vi "Smite.vi"(4 "Hook Search Path":path[](array[path]), 6 "Execute Hooks?":cluster{"Pre":bool, "Post":bool}={"Pre"=TRUE, "Post"=TRUE}, 8 "Error In":errorcluster, 10 "Graves":refnum<vi>[](array[refnum]), 11 "VI In":refnum<vi>) -> (0 "Error Out":errorcluster, 2 "Change Made?":bool, 3 "VI Out":refnum<vi>)   [LabVIEW 2018, in "Toolkit.lvlib"]
doc: "Changes zombies back into corpses at each grave. Disables the Corpse (legacy) frame and enables the Spirit (refactored) frame of each grave. A grave is Diagram Disable Structure with a RIP bookmark tag for its label, a.k.a. tombstone. No changes are made to any bookmarks or labels; only the enabled/disabled state of each frame is modified, but a Bookmark Info Change event is still fired."
uses:
  Toolkit.lvlib
  Typedefs/Grave Frames.ctl
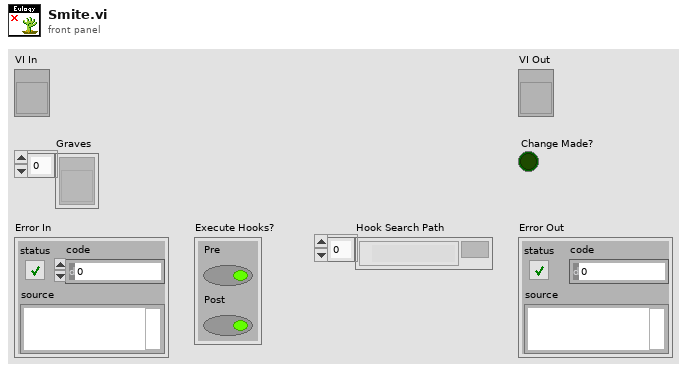
[diagram p1: front panel]
types:
  T1 = typedef "Toolkit.lvlib/Grave Frames.ctl" = enum16{"Corpse", "Spirit"}
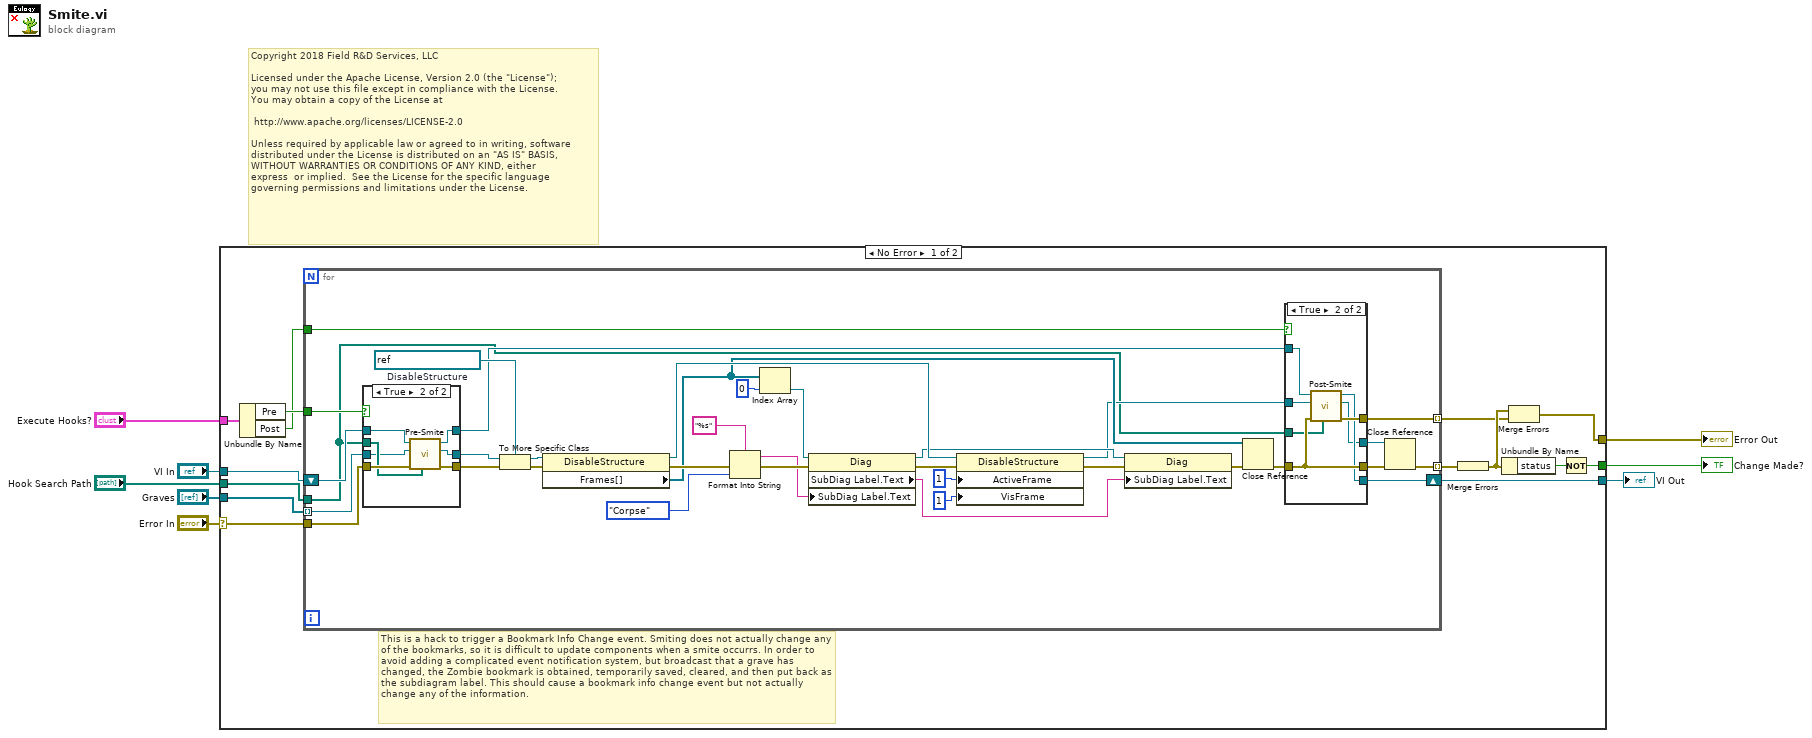
[diagram p0: block diagram]
diagram:
  # "Copyright 2018 Field R&D Services, LLC\n\nLicensed under the Apache License, Version 2.0 (the \"License\");\nyou may not use this file except in compliance with the License.\nYou may obtain a copy of the License at\n\n\thttp://www.apache.org/licenses/LICENSE-2.0\n\nUnless required by applicable law or agreed to in writing, software\ndistributed under the License is distributed on an \"AS IS\" BASIS,\nWITHOUT WARRANTIES OR CONDITIONS OF ANY KIND, either \nexpress  or implied.  See the License for the specific language \ngoverning permissions and limitations under the License."
  n1 = case shown="No Error" "Error In" {
    selector: "Error In" -> [w21 w79]
    tunnel: [w9 w79] -> w8
    tunnel: "Graves" -> [w22 _]
    tunnel: [w18 _] -> w5
    tunnel: "VI In" -> [w14 w78]
    tunnel: [w13 w78] -> w3
    tunnel: "Hook Search Path" -> [w12 _]
    tunnel: "Execute Hooks?" -> [w17 _]
    frame No Error {
      # "This is a hack to trigger a Bookmark Info Change event. Smiting does not actually change any of the bookmarks, so it is difficult to update components when a smite occurrs. In order to avoid adding a complicated event notification system, but broadcast that a grave has changed, the Zombie bookmark is obtained, temporarily saved, cleared, and then put back as the subdiagram label. This should cause a bookmark info change event but not actually change any of the information."
      n2 = Unbundle By Name(w17) -> ("Pre"=w16:bool, "Post"=w15:bool)
      n3 = for {
        tunnel: w22 -> [w36] mode=indexing
        tunnel: w21 -> [w37]
        tunnel: [w39] -> w20 mode=indexing
        tunnel: w16 -> [w38]
        tunnel: w15 -> [w25]
        shift-right: [w28] -> w13
        shift-left: w14 -> [w35]
        tunnel: w12 -> [w24]
        tunnel: [w23] -> w10 mode=indexing
        w57 = refnum<vi> refnum  # DisableStructure
        n4 = case shown="True" w38 {
          tunnel: w37 -> [w68 w77]
          tunnel: w36 -> [w69 w71]
          tunnel: w35 -> [w70 w74]
          tunnel: w24 -> [_ w75]
          tunnel: [w70 w73] -> w29
          tunnel: [w69 w72] -> w34
          tunnel: [w68 w76] -> w33
          frame False {
          }
          frame True {
            n5 = call "Pre-Smite.vi"("Search Path"=w75, "Error In"=w77, "Grave In"=w71, "VI In"=w74) -> ("Error Out"=w76:errorcluster, "Grave Out"=w72:refnum<vi>, "VI Out"=w73:refnum<vi>)  [unwired: 5 in]
          }
        }
        n6 = To More Specific Class(target class=w57, reference=w34, error in=w33) -> (specific class reference=w56:refnum<vi>, error out=w53:errorcluster)
        n7 = property class="DisableStructure"(reference=w56, error in=w53) -> (reference out=w43:refnum<vi>, error out=w50:errorcluster, "Frames[]"=w40:refnum<vi>[])
        n8 = Format Into String(format string="%s", error in=w50, Grave_Frames."Corpse" ("Frame")) -> (resulting string=w45:string, error out=w48:errorcluster)  [unwired: 1 in]
        n9 = Index Array(array=w40, index=0) -> (element=w51:refnum<vi>)
        n10 = property class="Diag"(reference=w51, error in=w48, "SubDiag Label.Text"=w45) -> (reference out=w42:refnum<vi>, error out=w49:errorcluster, "SubDiag Label.Text"=w41:string)
        n11 = property class="DisableStructure"(reference=w43, error in=w49, "ActiveFrame"=i16 1 ("Active Frame"), "VisFrame"=u32 1 ("Visible Frame")) -> (reference out=w27:refnum<vi>, error out=w44:errorcluster)
        n12 = property class="Diag"(reference=w42, error in=w44, "SubDiag Label.Text"=w41) -> (error out=w32:errorcluster)  [unwired: 1 out]
        n13 = Close Reference(reference=w40, error in (no error)=w32) -> (error out=w31:errorcluster)
        n14 = case shown="True" w25 {
          tunnel: w31 -> [w58 w66]
          tunnel: w27 -> [w59 w63]
          tunnel: w29 -> [w60 w64]
          tunnel: [w60 w65] -> w28
          tunnel: [w59 w62] -> w26
          tunnel: [w58 w66] -> w30
          tunnel: w24 -> [_ w61]
          tunnel: [_ w67] -> w23
          frame False {
          }
          frame True {
            n15 = call "Post-Smite.vi"("Search Path"=w61, "Error In"=w66, "Grave In"=w63, "VI In"=w64) -> ("Error Out"=w67:errorcluster, "Grave Out"=w62:refnum<vi>, "VI Out"=w65:refnum<vi>)  [unwired: 5 in]
          }
        }
        n16 = Close Reference(reference=w26, error in (no error)=w30) -> (error out=w39:errorcluster)
      }
      n17 = Merge Errors(w20) -> (w11:errorcluster)
      n18 = Unbundle By Name(w11) -> ("status"=w19:bool)
      n19 = Merge Errors(w11, w10) -> (w9:errorcluster)
      n20 = Not(x=w19) -> (.not. x?=w18:bool)
    }
    frame Error {
    }
  }
  "Error Out" <- w8
  "Change Made?" <- w5
  "VI Out" <- w3
